vi "Controller Apply PS Configuration.vi"(8 "Inverse PS Matrix Mapping":u32[][](array[numeric]), 9 "PS Configuration Status Out":refnum<notifier>, 10 "PS Configuration Status In":refnum<notifier>, 11 "Actuation Network In":T1) -> (2 "Maintain Config?":bool, 3 "Actuation Network Out":T1)   [LabVIEW 2011, in "Controller VIs.lvlib"]
uses:
  Controller VIs.lvlib
  Types Definitions/Type Actuation Network Configuration.ctl
  Type Definitions.lvlib
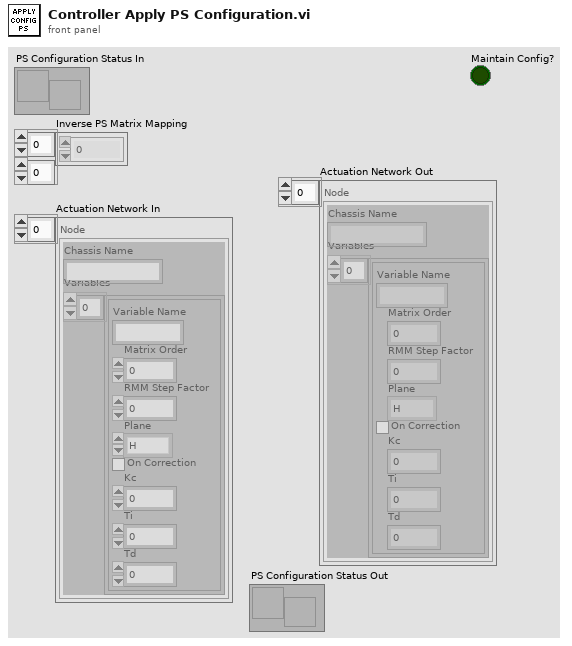
[diagram p1: front panel]
types:
  T1 = typedef "Type Definitions.lvlib/Type Actuation Network Configuration.ctl" = cluster{"Chassis Name":string, "Variables":cluster{"Variable Name":string, "Matrix Order":u32, "RMM Step Factor":dbl, "Plane":enum8{"H", "V"}, "On Correction":bool, "Kc":dbl, "Ti":dbl, "Td":dbl}[]}[]
  T2 = cluster{"Chassis Name":string, "Variables":cluster{"Variable Name":string, "Matrix Order":u32, "RMM Step Factor":dbl, "Plane":enum8{"H", "V"}, "On Correction":bool, "Kc":dbl, "Ti":dbl, "Td":dbl}[]}
  T3 = cluster{"Variable Name":string, "Matrix Order":u32, "RMM Step Factor":dbl, "Plane":enum8{"H", "V"}, "On Correction":bool, "Kc":dbl, "Ti":dbl, "Td":dbl}[]
  T4 = cluster{"Variable Name":string, "Matrix Order":u32, "RMM Step Factor":dbl, "Plane":enum8{"H", "V"}, "On Correction":bool, "Kc":dbl, "Ti":dbl, "Td":dbl}
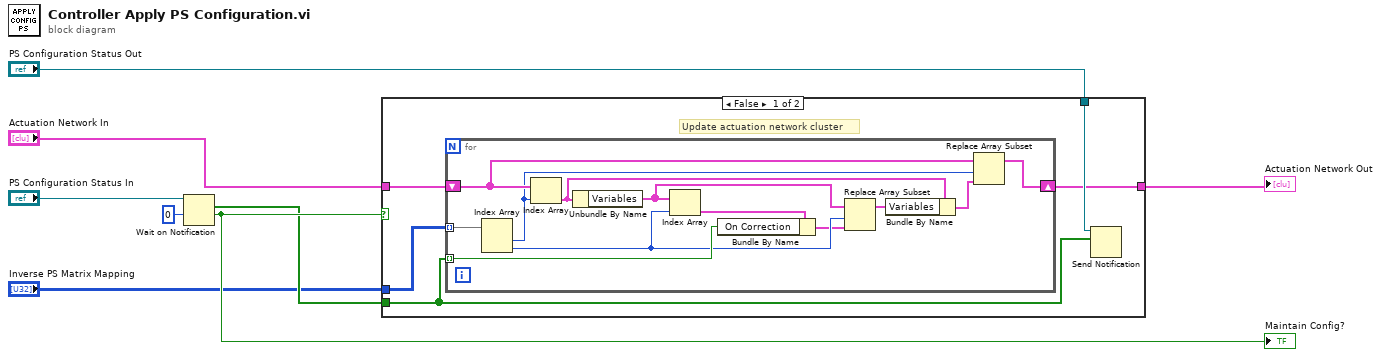
[diagram p0: block diagram]
diagram:
  n1 = Wait on Notification(notifier="PS Configuration Status In", timeout in ms (-1)=0) -> (notification=w3:bool[], timed out?=w5:bool)  [unwired: 2 in, 2 out]
  "Maintain Config?" <- w5
  n2 = case shown="False" w5 {
    tunnel: "Actuation Network In" -> [w12 w26]
    tunnel: [w11 w26] -> w7
    tunnel: "PS Configuration Status Out" -> [w13 _]
    tunnel: w3 -> [w9 _]
    tunnel: "Inverse PS Matrix Mapping" -> [w10 _]
    frame False {
      # "Update actuation network cluster"
      n3 = for {
        tunnel: w10 -> [w25] mode=indexing
        tunnel: w9 -> [w23] mode=indexing
        shift-right: [w14] -> w11
        shift-left: w12 -> [w22]
        n4 = Index Array(array=w25) -> (element #1=w21:u32, element #2=w19:u32)  [unwired: 2 in]
        n5 = Index Array(array=w22, index=w21) -> (element=w17:T2)
        n6 = Unbundle By Name(w17) -> ("Variables"=w20:T3)
        n7 = Index Array(array=w20, index=w19) -> (element=w24:T4)
        n8 = Bundle By Name(cluster=w24, "On Correction"=w23) -> (w18:T4)
        n9 = Replace Array Subset(array=w20, new element=w18, index=w19) -> (w16:T3)
        n10 = Bundle By Name(cluster=w17, "Variables"=w16) -> (w15:T2)
        n11 = Replace Array Subset(array=w22, new element=w15, index=w21) -> (w14:T1)
      }
      n12 = Send Notification(notification=w9, notifier=w13) -> ()  [unwired: 1 in, 2 out]
    }
    frame True {
    }
  }
  "Actuation Network Out" <- w7
